vi "XIPIN_ILA_(Integrated_Logic_Analyzer)_6_0.vi"   [LabVIEW 2017]
doc: "The Integrated Logic Analyzer (ILA) core is a customizable logic analyzer core that can be used to monitor any internal signal of your design. The ILA core includes many advanced features of modern logic analyzers, including Boolean trigger equations, customizable data capture buffer depth, and optional trigger input/output ports. Because the ILA core is synchronous to the design being monitored, all design clock constraints that are applied to your design are also applied to the components inside the ILA core. Run-time interaction with this core requires the use of the Vivado logic analyzer feature.\n------------------------------------\n<b>Need License</b> : No\n<b>Interface</b> : AXI4 AXI4-Stream"
uses:
  <vilib>/rvi/XilinxIP/XIPIN_XNode/niFpgaXIPIN.xnode
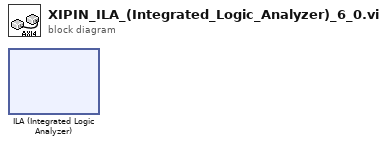
[diagram p0: block diagram]
diagram:
  n1 = xnode ("ILA (Integrated Logic Analyzer)")() -> ()
